vi "Msg.vi"(7 "jettl in":refnum<class "jettl.lvclass">, 11 "Queue Create Msg Strategy in":refnum<class "Queue Create Msg Strategy.lvclass">) -> (5 "jettl out":refnum<class "jettl.lvclass">)   [LabVIEW 2021, in "jettl.lvlib" / "Queue Create.lvlib" / "Queue Create Msg Strategy.lvclass"]
uses:
  Queue Create Msg Strategy.lvclass
  jettl/jettl.lvclass
  Queue Create/Queue Create.lvclass
  Queue Create Msg Strategy.lvclass/Queue Create Msg Strategy.ctl
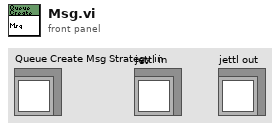
[diagram p1: front panel]
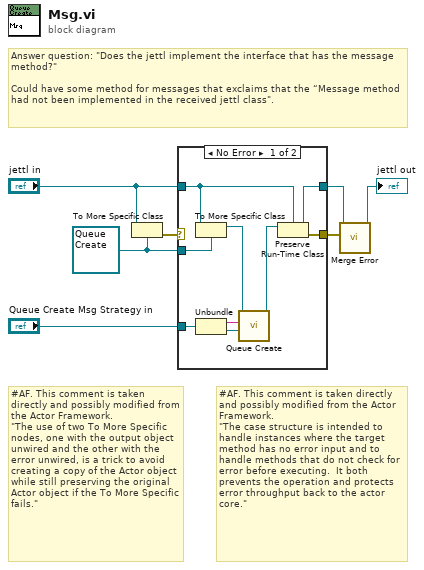
[diagram p0: block diagram]
diagram:
  w6 = refnum<class "Queue Create.lvclass"> refnum ("Create.lvlib:Create.lvclass")
  # "#AF. This comment is taken directly and possibly modified from the Actor Framework.\n\"The use of two To More Specific nodes, one with the output object unwired and the other with the error unwired, is a trick to avoid creating a copy of the Actor object while still preserving the original Actor object if the To More Specific fails.\""
  # "#AF. This comment is taken directly and possibly modified from the Actor Framework.\n\"The case structure is intended to handle instances where the target method has no error input and to handle methods that do not check for error before executing.  It both prevents the operation and protects error throughput back to the actor core.\""
  # "Answer question: \"Does the jettl implement the interface that has the message method?\"\n\nCould have some method for messages that exclaims that the “Message method had not been implemented in the received jettl class\"."
  n1 = To More Specific Class(target class=w6, reference="jettl in") -> (error out=w7:errorcluster)  [unwired: 1 in, 1 out]
  n2 = case shown="No Error" w7 {
    selector: w7 -> [_ w17]
    tunnel: [w11 w18] -> w3
    tunnel: "jettl in" -> [w12 w18]
    tunnel: w6 -> [w16 _]
    tunnel: "Queue Create Msg Strategy in" -> [w15 _]
    tunnel: [w10 w17] -> w4
    frame No Error {
      n3 = To More Specific Class(target class=w16, reference=w12) -> (specific class reference=w9:refnum<class "Queue Create.lvclass">)  [unwired: 1 in, 1 out]
      n4 = Unbundle(w15) -> (w14:string, w13:refnum<class "Queue jettl.lvclass">)
      n5 = call-dynamic "Queue Create.vi"("Queue jettl"=w13, "Alias"=w14, "Queue Create in"=w9) -> ("Queue Create out"=w8:refnum<class "Queue Create.lvclass">)  [unwired: 8 in]
      n6 = Preserve Run-Time Class(object in=w8, 2:w12) -> (object out=w11:refnum<class "jettl.lvclass">, error out=w10:errorcluster)  [unwired: 1 in]
    }
    frame Error {
    }
  }
  n7 = call-dynamic "Merge Error.vi"("Error"=w4, "Merge Error in"=w3) -> ("Merge Error out"=→"jettl out":refnum<class "jettl.lvclass">)  [unwired: 9 in]
